vi "Lab 2.vi"() -> ()   [LabVIEW 2014]
panel:
  out "Random Number Generated":dbl
  out "Result":dbl
  in  "B":dbl
  in  "A":dbl
  in  "Function":u8(slide) scale=0.0..5.0
  out "y":dbl
  in  "c":dbl
  in  "x":dbl
  in  "m":dbl
  in  "y=mx2+c or\ny=mx+c":bool
  in  "Temperature":dbl
  in  "True / False":bool
  out "Converted Temperature":dbl
  in  "Stop Button":bool
  out "Fahrenheit (F)":dbl
  in  "Celsius (C)":dbl
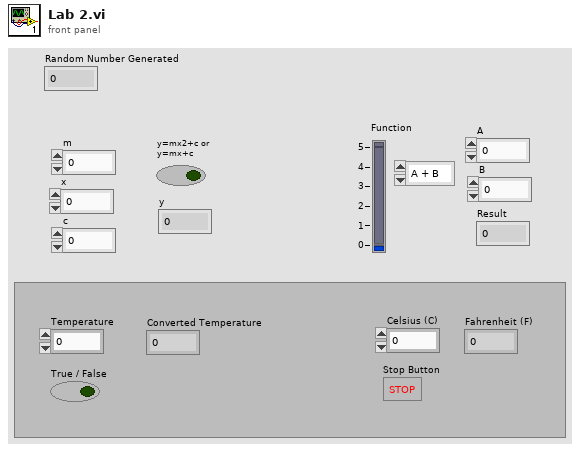
[diagram p1: front panel]
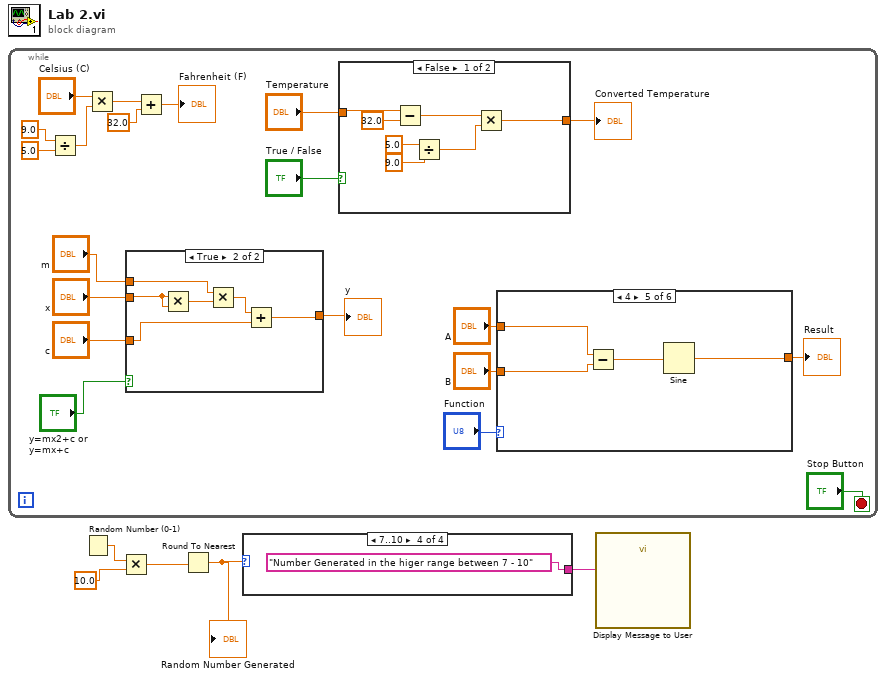
[diagram p0: block diagram]
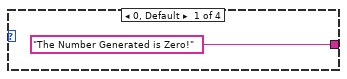
[diagram p2: hidden frame]
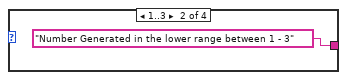
[diagram p3: hidden frame]
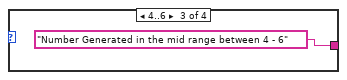
[diagram p4: hidden frame]
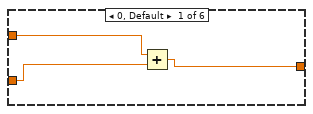
[diagram p5: hidden frame]
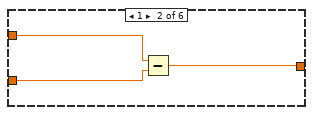
[diagram p6: hidden frame]
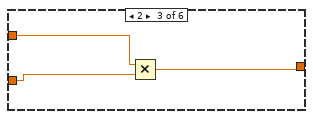
[diagram p7: hidden frame]
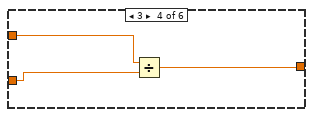
[diagram p8: hidden frame]
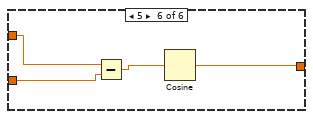
[diagram p9: hidden frame]
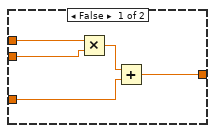
[diagram p10: hidden frame]
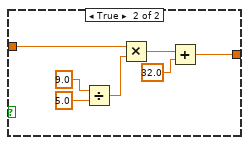
[diagram p11: hidden frame]
diagram:
  n1 = while {
    stop <- "Stop Button" stop-if-true
    n2 = Divide(x=9.0, y=5.0) -> (x/y=w23:dbl)
    n3 = Multiply(x="Celsius (C)", y=w23) -> (x*y=w21:dbl)
    n4 = case shown="True" "y=mx2+c or\ny=mx+c" {
      tunnel: "m" -> [w50 w51]
      tunnel: "x" -> [w49 w53]
      tunnel: "c" -> [w47 w55]
      tunnel: [w46 w54] -> w10
      frame False {
        n5 = Multiply(x=w50, y=w49) -> (x*y=w48:dbl)
        n6 = Add(x=w48, y=w47) -> (x+y=w46:dbl)
      }
      frame True {
        n7 = Multiply(x=w53, y=w53) -> (x*y=w52:dbl)
        n8 = Multiply(x=w51, y=w52) -> (x*y=w56:dbl)
        n9 = Add(x=w56, y=w55) -> (x+y=w54:dbl)
      }
    }
    "y" <- w10
    n10 = Add(x=w21, y=32.0) -> (x+y=→"Fahrenheit (F)":dbl)
    n11 = case shown="False" "True / False" {
      tunnel: [w63 w65] -> w17
      tunnel: "Temperature" -> [w62 w64]
      frame False {
        n12 = Subtract(x=w62, y=32.0) -> (x-y=w60:dbl)
        n13 = Divide(x=5.0, y=9.0) -> (x/y=w57:dbl)
        n14 = Multiply(x=w60, y=w57) -> (x*y=w63:dbl)
      }
      frame True {
        n15 = Divide(x=9.0, y=5.0) -> (x/y=w68:dbl)
        n16 = Multiply(x=w64, y=w68) -> (x*y=w67:dbl)
        n17 = Add(x=w67, y=32.0) -> (x+y=w65:dbl)
      }
    }
    "Converted Temperature" <- w17
    n18 = case shown="4" "Function" {
      tunnel: "A" -> [w28 w31 w34 w37 w40 w44]
      tunnel: "B" -> [w27 w29 w33 w36 w39 w43]
      tunnel: [w26 w30 w32 w35 w38 w42] -> w6
      frame 0, Default {
        n19 = Add(x=w28, y=w27) -> (x+y=w26:dbl)
      }
      frame 1 {
        n20 = Subtract(x=w31, y=w29) -> (x-y=w30:dbl)
      }
      frame 2 {
        n21 = Multiply(x=w34, y=w33) -> (x*y=w32:dbl)
      }
      frame 3 {
        n22 = Divide(x=w37, y=w36) -> (x/y=w35:dbl)
      }
      frame 4 {
        n23 = Subtract(x=w40, y=w39) -> (x-y=w41:dbl)
        n24 = Sine(x=w41) -> (sin(x)=w38:dbl)
      }
      frame 5 {
        n25 = Subtract(x=w44, y=w43) -> (x-y=w45:dbl)
        n26 = Cosine(x=w45) -> (cos(x)=w42:dbl)
      }
    }
    "Result" <- w6
  }
  n27 = Random Number (0-1)() -> (number: 0 to 1=w5:dbl)
  n28 = Multiply(x=w5, y=10.0) -> (x*y=w3:dbl)
  n29 = Round To Nearest(number=w3) -> (nearest integer value=w2:dbl)
  "Random Number Generated" <- w2
  n30 = case shown="7..10" w2 {
    tunnel: ["The Number Generated is Zero!" "Number Generated in the lower range between 1 - 3" "Number Generated in the mid range between 4 - 6" "Number Generated in the higer range between 7 - 10"] -> w1
    frame 0, Default {
    }
    frame 1..3 {
    }
    frame 4..6 {
    }
    frame 7..10 {
    }
  }
  n31 = call "Display Message to User"("Message"=w1) -> ()  [unwired: 9 in, 2 out]
